vi "JSON Escape.vi"(1 "JSON String":string) -> (0 "Escaped JSON String":string)   [LabVIEW 2013, in "LV JSON.lvlib"]
uses:
  LV JSON.lvlib
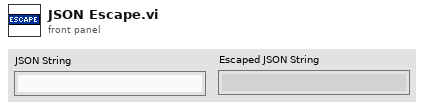
[diagram p1: front panel]
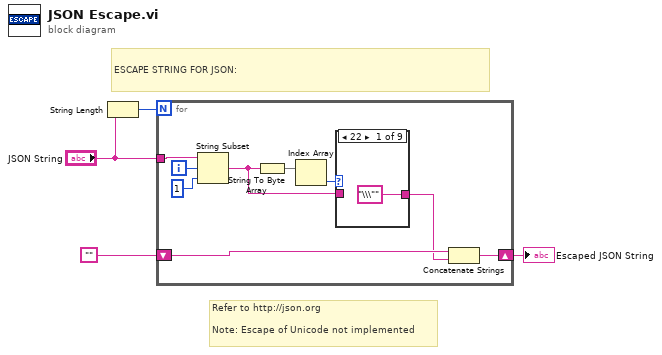
[diagram p0: block diagram]
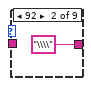
[diagram p2: hidden frame]
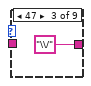
[diagram p3: hidden frame]
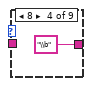
[diagram p4: hidden frame]
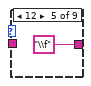
[diagram p5: hidden frame]
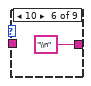
[diagram p6: hidden frame]
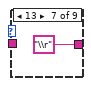
[diagram p7: hidden frame]
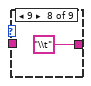
[diagram p8: hidden frame]
diagram:
  # "ESCAPE STRING FOR JSON:"
  # "Refer to http://json.org\n\nNote: Escape of Unicode not implemented"
  n1 = String Length(string="JSON String") -> (length=w3:i32)
  n2 = for {
    N: w3 -> [_]
    shift-right: [w8] -> w1
    shift-left: "" -> [w10]
    tunnel: "JSON String" -> [w11]
    i -> [w13]
    n3 = String Subset(string=w11, offset (0)=w13, length (rest)=1 ("length (rest)")) -> (substring=w5:string)
    n4 = String To Byte Array(string=w5) -> (unsigned byte array=w7:u8[])
    n5 = Index Array(array=w7) -> (element=w6:u8)  [unwired: 1 in]
    n6 = case shown="22" w6 {
      tunnel: ["\\\"" "\\\\" "\\/" "\\b" "\\f" "\\n" "\\r" "\\t" w22] -> w9
      tunnel: w5 -> [_ _ _ _ _ _ _ _ w22]
      frame 34 {
      }
      frame 92 {
      }
      frame 47 {
      }
      frame 8 {
      }
      frame 12 {
      }
      frame 10 {
      }
      frame 13 {
      }
      frame 9 {
      }
      frame Default {
      }
    }
    n7 = Concatenate Strings(w10, w9) -> (w8:string)
  }
  "Escaped JSON String" <- w1
